vi "Select Spectra.vi"(8 "error in (no error)":errorcluster, 10 "Selector Input":bool[](array[boolean]), 11 "All Spectra":cluster{"f0":dbl, "df":dbl, "magnitude":dbl[]}[](array[cluster])) -> (0 "error out":errorcluster, 3 "Selected Spectra":cluster{"f0":dbl, "df":dbl, "magnitude":dbl[]}[](array[cluster]))   [LabVIEW 2013]
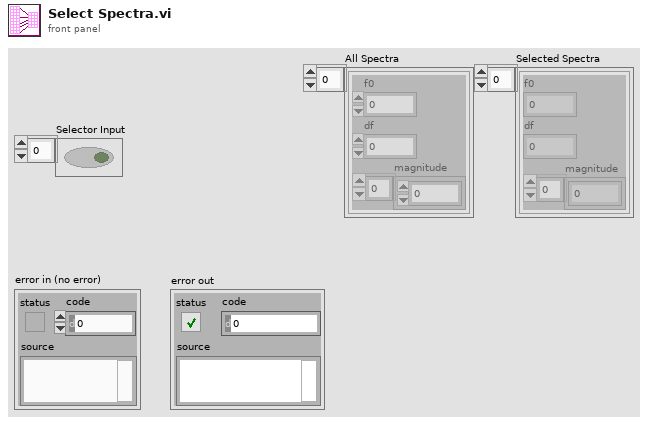
[diagram p1: front panel]
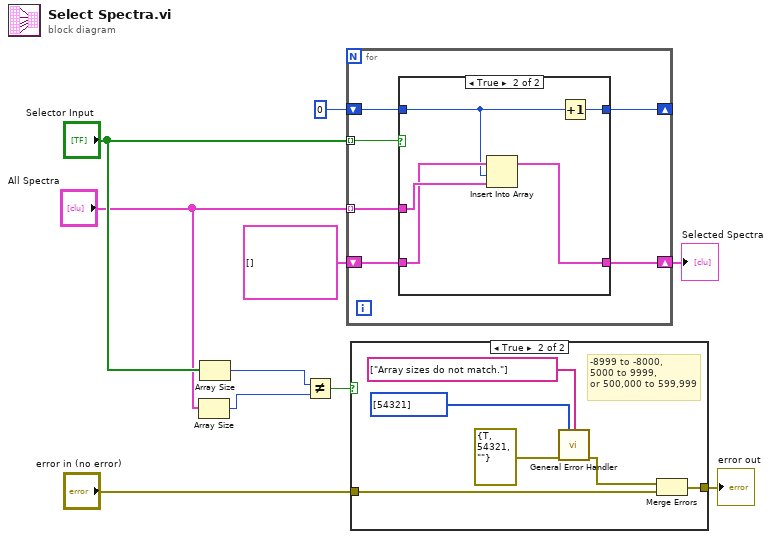
[diagram p0: block diagram]
diagram:
  n1 = Array Size(array="All Spectra") -> (size(s)=w2:i32)
  n2 = Array Size(array="Selector Input") -> (size(s)=w8:i32)
  n3 = Not Equal?(x=w8, y=w2) -> (x != y?=w7:bool)
  n4 = for {
    tunnel: "All Spectra" -> [w15] mode=indexing
    tunnel: "Selector Input" -> [w16] mode=indexing
    shift-right: [w12] -> w3
    shift-left: cluster{"f0":dbl, "df":dbl, "magnitude":dbl[]}[] [] -> [w14]
    shift-right: [w11] -> _
    shift-left: 0 -> [w13]
    n5 = case shown="True" w16 {
      tunnel: w15 -> [_ w23]
      tunnel: w14 -> [w18 w22]
      tunnel: w13 -> [w17 w20]
      tunnel: [w18 w21] -> w12
      tunnel: [w17 w19] -> w11
      frame False {
      }
      frame True {
        n6 = Insert Into Array(array=w22, index=w20, new element=w23) -> (w21:cluster{"f0":dbl, "df":dbl, "magnitude":dbl[]}[])
        n7 = Increment(x=w20) -> (x+1=w19:i32)
      }
    }
  }
  "Selected Spectra" <- w3
  n8 = case shown="True" w7 {
    tunnel: "error in (no error)" -> [w24 w26]
    tunnel: [w24 w27] -> w5
    frame False {
    }
    frame True {
      # "-8999 to -8000,\n5000 to 9999,\nor 500,000 to 599,999"
      n9 = call <vilib>:"General Error Handler.vi"("[user-defined codes]"=i32[] [54321], "[user-defined descriptions]"=string[] ["Array sizes do not match."], "error in (no error)"=errorcluster {"status"=TRUE, "code"=54321, "source"=""}) -> ("error out"=w25:errorcluster)  [unwired: 8 in, 4 out]
      n10 = Merge Errors(w25, w26) -> (w27:errorcluster)
    }
  }
  "error out" <- w5
